vi "Begin.vi"() -> (0 "error out":errorcluster)   [LabVIEW 2013]
doc: "Called before other user functions, this VI is expected to open initial I/O refnums, load in file data, and do all program initialization. Notice that the <B>error out</B> terminal is simply used for data flow. Wiring it to other structures or subVIs ensures that this VI runs first."
uses:
  <vilib>/Rock Robotics/WPI/DriverStation/WPI_DriverStationRobotMode2.ctl
  <vilib>/Rock Robotics/WPI/Joystick/WPI_JoystickDeviceEnum.ctl
  <vilib>/Rock Robotics/SystemInterfaces/DIO/FPGA_DIOPWMChannel.ctl
  <vilib>/Rock Robotics/SystemInterfaces/AI/FPGA_AIGyroChannel.ctl
  <vilib>/Rock Robotics/SystemInterfaces/Typedef/FPGA_TypedefAnalogModuleForGyro.ctl
  <vilib>/Rock Robotics/SystemInterfaces/DIO/FPGA_DIOChannel.ctl
  <vilib>/Rock Robotics/SystemInterfaces/AI/FPGA_AIChannel.ctl
  <vilib>/Rock Robotics/SystemInterfaces/Typedef/FPGA_TypedefAnalogModule.ctl
  <vilib>/Rock Robotics/SystemInterfaces/DIO/FPGA_DIORelayChannel.ctl
  <vilib>/Rock Robotics/SystemInterfaces/Typedef/FPGA_TypedefDigitalModule.ctl
  Robot Global Data.vi
  <vilib>/Rock Robotics/WPI/MotorControl/WPI_MotorControlOpen Talon.vi
panel:
  out "error out 3":errorcluster
  out "error out 2":errorcluster
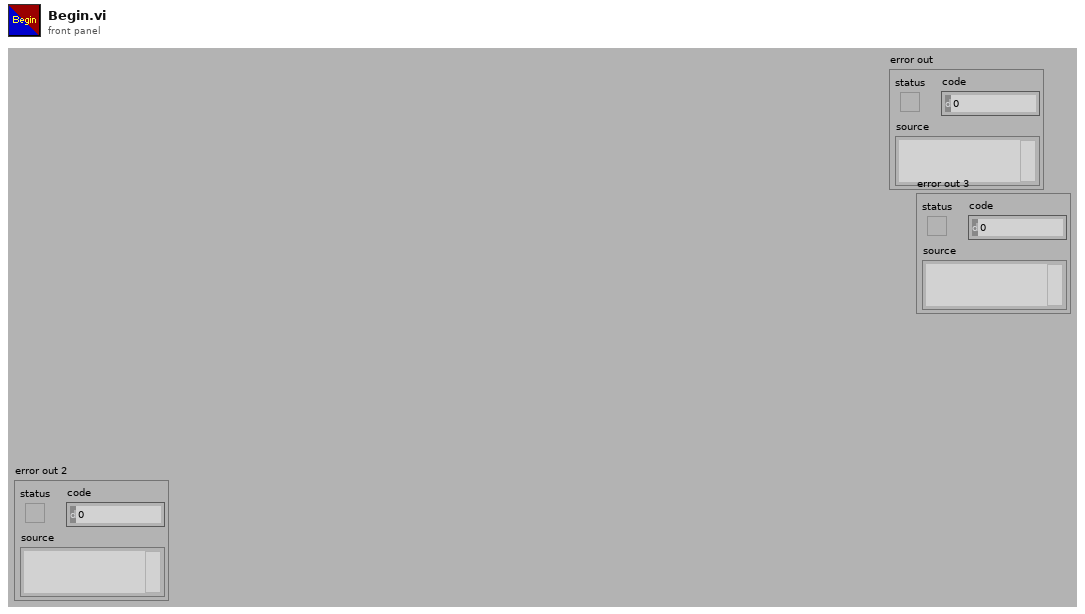
[diagram p1: front panel]
types:
  T1 = typedef "FPGA_TypedefDigitalModule.ctl" = enum16{"Digital Module 1", "Digital Module 2"}
  T2 = typedef "FPGA_DIORelayChannel.ctl" = enum8{"Relay 1", "Relay 2", "Relay 3", "Relay 4", "Relay 5", "Relay 6", "Relay 7", "Relay 8", "Invalid"}
  T3 = typedef "FPGA_DIOChannel.ctl" = enum8{"DIO 1", "DIO 2", "DIO 3", "DIO 4", "DIO 5", "DIO 6", "DIO 7", "DIO 8", "DIO 9", "DIO 10", "DIO 11", "DIO 12", "DIO 13", "DIO 14", "Invalid"}
  T4 = typedef "FPGA_DIOPWMChannel.ctl" = enum8{"PWM 1", "PWM 2", "PWM 3", "PWM 4", "PWM 5", "PWM 6", "PWM 7", "PWM 8", "PWM 9", "PWM 10", "Invalid"}
  T5 = typedef "FPGA_TypedefAnalogModule.ctl" = enum16{"Analog Module 1", "Analog Module 2"}
  T6 = typedef "FPGA_AIChannel.ctl" = enum8{"AI 1", "AI 2", "AI 3", "AI 4", "AI 5", "AI 6", "AI 7", "AI 8", "Invalid"}
  T7 = typedef "WPI_JoystickDeviceEnum.ctl" = enum16{"USB 1", "USB 2", "USB 3", "USB 4", "Kinect 1", "Kinect 2"}
  T8 = typedef "FPGA_TypedefAnalogModuleForGyro.ctl" = enum16{"Analog Module 1"}
  T9 = typedef "FPGA_AIGyroChannel.ctl" = enum8{"AI 1", "AI 2", "Invalid"}
  T10 = typedef "WPI_DriverStationRobotMode2.ctl" = enum16{"Autonomous Disabled", "Autonomous Enabled", "Teleop Disabled", "Teleop Enabled", "Timeout", "Finish", "Test Disabled", "Test Enabled"}
  T11 = typedef "WPI_JoystickDevRef.ctl" = cluster{"Device":T7}
  T12 = typedef "WPI_ServoDeviceRef.ctl" = cluster{"DeviceStatus":errorcluster, "Digital Module":T1, "PWM Channel":T4, "DeadBand":T13}
  T13 = typedef "WPI_PWMDeadband.ctl" = cluster{"Name":string, "maxPositivePwm":i32, "minPositivePwm":i32, "centerPwm":i32, "maxNegativePwm":i32, "minNegativePwm":i32, "angularRange":u16}
  T14 = typedef "WPI_MotorControlDeviceRef.ctl" = cluster{"DeviceStatus":errorcluster, "Type":enum16{"PWM", "CAN"}, "PWM":cluster{"Digital Module":T1, "PWM Channel":T4, "DeadBand":T13}, "CAN":cluster{"Device Number":u8, "Control Mode":T15, "Semaphore":T16, "Max Vout":dbl}, "Invert":bool, "TransformRef":T17, "InvTransformRef":T17}
  T15 = typedef "WPI_CANJaguar_ControlMode.ctl" = enum8{"Percent VBus", "Current", "Speed", "Position", "Voltage"}
  T16 = typedef "Semaphore RefNum" = refnum<k1>
  T17 = typedef "WPI_PWMTransform_ConPane.ctl" = refnum<vi>
  T18 = typedef "WPI_RelayDevRef.ctl" = cluster{"DevStatus":errorcluster, "Relay Channel":T2, "Digital Module":T1, "Relay Direction":T19}
  T19 = typedef "WPI_RelayDirection.ctl" = enum16{"Both directions", "Forward only", "Reverse only"}
  T20 = typedef "WPI_DigitalInputDevRef.ctl" = cluster{"DevStatus":errorcluster, "DIO Channel":T3, "Digital Module":T1}
  T21 = typedef "WPI_AnalogChannelDevRef.ctl" = cluster{"DevStatus":errorcluster, "Analog Module":T5, "Analog Channel":T6}
  T22 = typedef "WPI_GyroDevRef.ctl" = cluster{"DevStatus":errorcluster, "Analog Module":T5, "Analog Channel":T6, "Offset":dbl, "Gain (VoltsPerDegree/Second)":dbl}
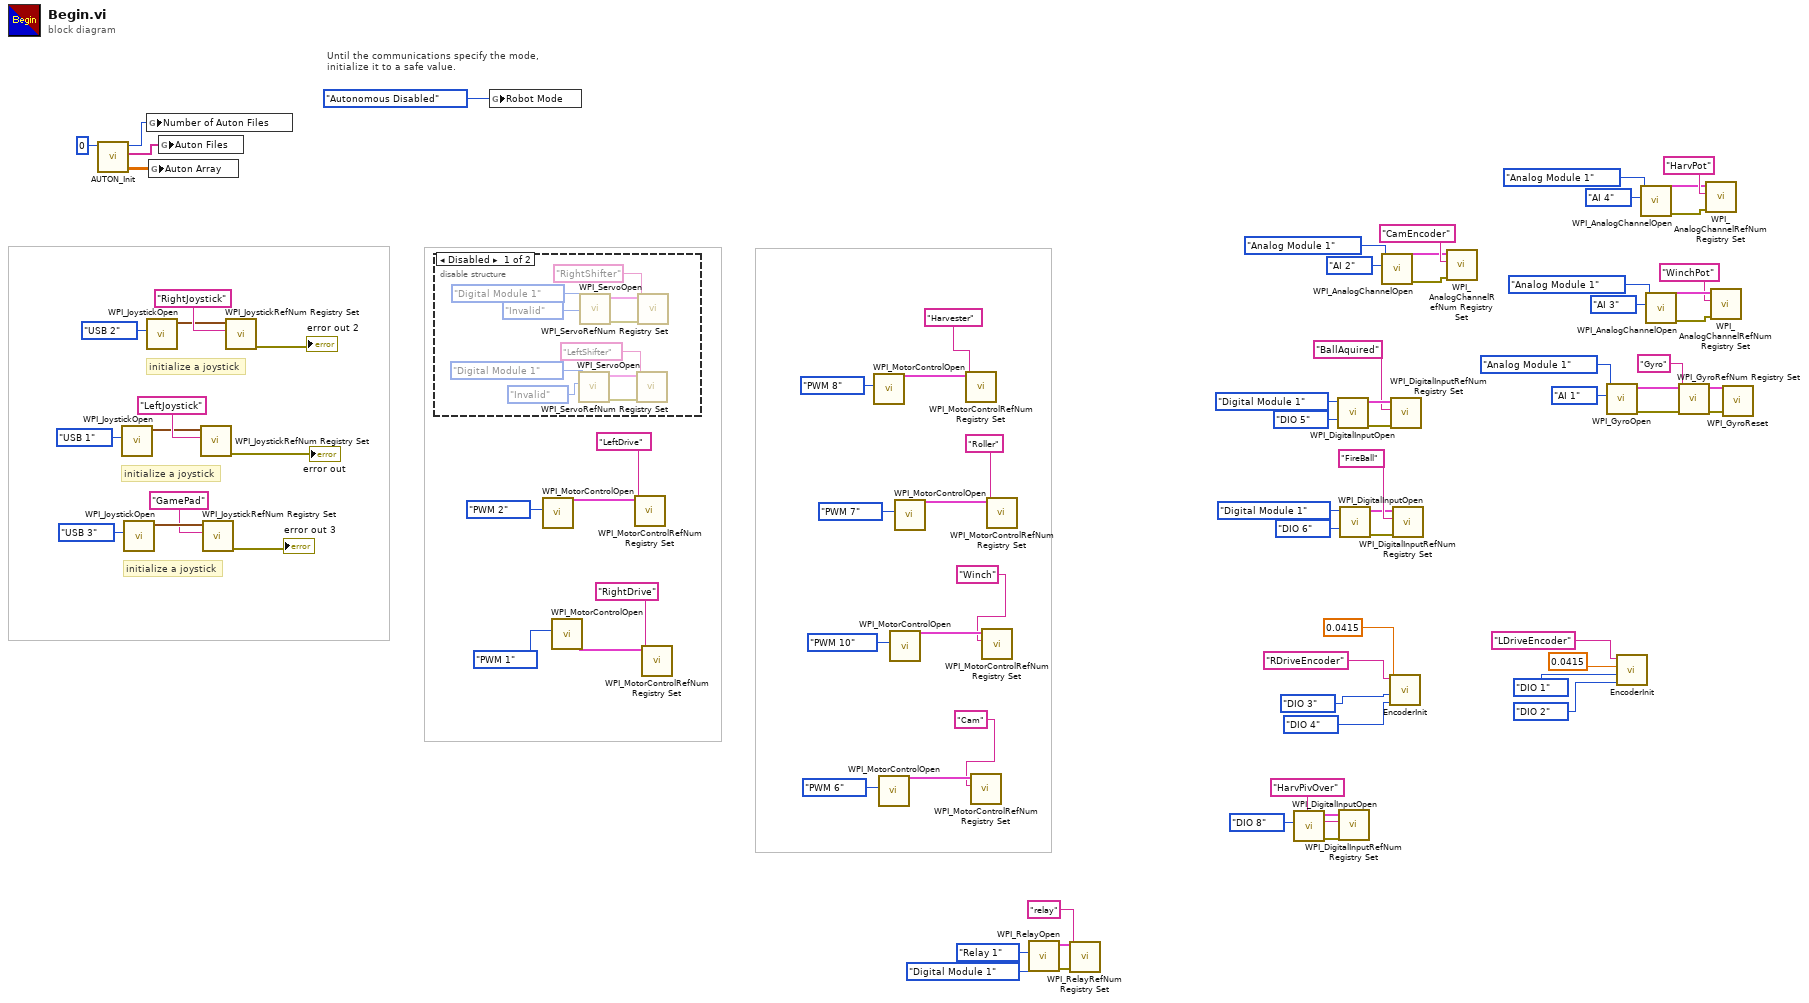
[diagram p0: block diagram]
diagram:
  # "initialize a joystick"
  # "initialize a joystick"
  # "initialize a joystick"
  # "Until the communications specify the mode,\ninitialize it to a safe value."
  n1 = call "AUTON_Init.vi"("Default File"=0) -> ("Auton Array"=w68:dbl[][], "Auton Files"=w67:string[], "Number of Auton Files"=w66:i64)  [unwired: 8 in]
  n2 = call <vilib>:"WPI_JoystickOpen.vi"("JoystickDevice"=WPI_JoystickDeviceEnum."USB 1") -> ("JoystickDevRef"=w82:T11)  [unwired: 10 in]
  n3 = call <vilib>:"WPI_JoystickOpen.vi"("JoystickDevice"=WPI_JoystickDeviceEnum."USB 3") -> ("JoystickDevRef"=w46:T11)  [unwired: 10 in]
  n4 = global write "Robot Global Data.vi" "Number of Auton Files"(w66) -> ()
  n5 = call <vilib>:"WPI_JoystickOpen.vi"("JoystickDevice"=WPI_JoystickDeviceEnum."USB 2") -> ("JoystickDevRef"=w78:T11)  [unwired: 10 in]
  n6 = global write "Robot Global Data.vi" "Auton Array"(w68) -> ()
  n7 = global write "Robot Global Data.vi" "Auton Files"(w67) -> ()
  n8 = call <vilib>:"WPI_JoystickRefNum Registry Set.vi"("refnum name"="LeftJoystick", "JoystickDevRef"=w82) -> ("error out"=→"error out":errorcluster)  [unwired: 8 in, 1 out]
  n9 = call <vilib>:"WPI_JoystickRefNum Registry Set.vi"("refnum name"="GamePad", "JoystickDevRef"=w46) -> ("error out"=→"error out 3":errorcluster)  [unwired: 8 in, 1 out]
  n10 = call <vilib>:"WPI_JoystickRefNum Registry Set.vi"("refnum name"="RightJoystick", "JoystickDevRef"=w78) -> ("error out"=→"error out 2":errorcluster)  [unwired: 8 in, 1 out]
  n11 = disable-structure shown="Disabled" {
    frame Disabled {
      n12 = call <vilib>:"WPI_ServoOpen.vi"("PWM Channel"=FPGA_DIOPWMChannel."Invalid", "Digital Module (Module 1)"=FPGA_TypedefDigitalModule."Digital Module 1") -> ("error out"=w94:errorcluster, "ServoDeviceRef"=w87:T12)  [unwired: 8 in]
      n13 = call <vilib>:"WPI_ServoOpen.vi"("PWM Channel"=FPGA_DIOPWMChannel."Invalid", "Digital Module (Module 1)"=FPGA_TypedefDigitalModule."Digital Module 1") -> ("error out"=w93:errorcluster, "ServoDeviceRef"=w92:T12)  [unwired: 8 in]
      n14 = call <vilib>:"WPI_ServoRefNum Registry Set.vi"("error in (no error)"=w94, "refnum name"="LeftShifter", "ServoDeviceRef"=w87) -> ()  [unwired: 7 in, 2 out]
      n15 = call <vilib>:"WPI_ServoRefNum Registry Set.vi"("error in (no error)"=w93, "refnum name"="RightShifter", "ServoDeviceRef"=w92) -> ()  [unwired: 7 in, 2 out]
    }
    frame Enabled {
    }
  }
  n16 = global write "Robot Global Data.vi" "Robot Mode"(WPI_DriverStationRobotMode2."Autonomous Disabled" ("Robot Mode")) -> ()
  n17 = call-poly <vilib>:"WPI_MotorControlOpen.vi"("PWM Channel"=FPGA_DIOPWMChannel."PWM 2") -> ("MotorControlDeviceRef"=w74:T14)  [unwired: 9 in, 1 out]
  n18 = call-poly <vilib>:"WPI_MotorControlOpen.vi"("PWM Channel"=FPGA_DIOPWMChannel."PWM 1") -> ("MotorControlDeviceRef"=w71:T14)  [unwired: 9 in, 1 out]
  n19 = call <vilib>:"WPI_MotorControlRefNum Registry Set.vi"("refnum name"="LeftDrive", "MotorControlDevRef"=w74) -> ()  [unwired: 8 in, 2 out]
  n20 = call <vilib>:"WPI_MotorControlRefNum Registry Set.vi"("refnum name"="RightDrive", "MotorControlDevRef"=w71) -> ()  [unwired: 8 in, 2 out]
  n21 = call-poly <vilib>:"WPI_MotorControlOpen.vi"("PWM Channel"=FPGA_DIOPWMChannel."PWM 8") -> ("MotorControlDeviceRef"=w64:T14)  [unwired: 9 in, 1 out]
  n22 = call-poly <vilib>:"WPI_MotorControlOpen.vi"("PWM Channel"=FPGA_DIOPWMChannel."PWM 6") -> ("MotorControlDeviceRef"=w28:T14)  [unwired: 9 in, 1 out]
  n23 = call-poly <vilib>:"WPI_MotorControlOpen.vi"("PWM Channel"=FPGA_DIOPWMChannel."PWM 10") -> ("MotorControlDeviceRef"=w30:T14)  [unwired: 9 in, 1 out]
  n24 = call-poly <vilib>:"WPI_MotorControlOpen.vi"("PWM Channel"=FPGA_DIOPWMChannel."PWM 7") -> ("MotorControlDeviceRef"=w62:T14)  [unwired: 9 in, 1 out]
  n25 = call <vilib>:"WPI_MotorControlRefNum Registry Set.vi"("refnum name"="Harvester", "MotorControlDevRef"=w64) -> ()  [unwired: 8 in, 2 out]
  n26 = call <vilib>:"WPI_MotorControlRefNum Registry Set.vi"("refnum name"="Cam", "MotorControlDevRef"=w28) -> ()  [unwired: 8 in, 2 out]
  n27 = call <vilib>:"WPI_MotorControlRefNum Registry Set.vi"("refnum name"="Winch", "MotorControlDevRef"=w30) -> ()  [unwired: 8 in, 2 out]
  n28 = call <vilib>:"WPI_MotorControlRefNum Registry Set.vi"("refnum name"="Roller", "MotorControlDevRef"=w62) -> ()  [unwired: 8 in, 2 out]
  n29 = call <vilib>:"WPI_RelayOpen.vi"("Relay Channel"=FPGA_DIORelayChannel."Relay 1", "Digital Module (Module 1)"=FPGA_TypedefDigitalModule."Digital Module 1") -> ("error out"=w4:errorcluster, "RelayDevRef"=w3:T18)  [unwired: 8 in]
  n30 = call <vilib>:"WPI_RelayRefNum Registry Set.vi"("error in (no error)"=w4, "refnum name"="relay", "RelayDevRef"=w3) -> ()  [unwired: 7 in, 2 out]
  n31 = call <vilib>:"WPI_DigitalInputOpen.vi"("DIO Channel"=FPGA_DIOChannel."DIO 8") -> ("error out"=w32:errorcluster, "DigitalInputDevRef"=w33:T20)  [unwired: 9 in]
  n32 = call <vilib>:"WPI_DigitalInputOpen.vi"("DIO Channel"=FPGA_DIOChannel."DIO 5", "Digital Module (Module 1)"=FPGA_TypedefDigitalModule."Digital Module 1") -> ("error out"=w56:errorcluster, "DigitalInputDevRef"=w55:T20)  [unwired: 8 in]
  n33 = call <vilib>:"WPI_DigitalInputRefNum Registry Set.vi"("error in (no error)"=w32, "refnum name"="HarvPivOver", "DigitalInputDevRef"=w33) -> ()  [unwired: 7 in, 2 out]
  n34 = call <vilib>:"WPI_DigitalInputOpen.vi"("DIO Channel"=FPGA_DIOChannel."DIO 6", "Digital Module (Module 1)"=FPGA_TypedefDigitalModule."Digital Module 1") -> ("error out"=w16:errorcluster, "DigitalInputDevRef"=w17:T20)  [unwired: 8 in]
  n35 = call <vilib>:"WPI_AnalogChannelOpen.vi"("Analog Channel"=FPGA_AIChannel."AI 2", "Analog Module (Module 1)"=FPGA_TypedefAnalogModule."Analog Module 1") -> ("error out"=w22:errorcluster, "AIDeviceRef"=w21:T21)  [unwired: 8 in]
  n36 = call "EncoderInit.vi"("refnum name"="RDriveEncoder", "DistancePerCount"=0.0415, "DIO Channel"=FPGA_DIOChannel."DIO 3", "DIO Channel 2"=FPGA_DIOChannel."DIO 4") -> ()  [unwired: 7 in]
  n37 = call <vilib>:"WPI_DigitalInputRefNum Registry Set.vi"("error in (no error)"=w56, "refnum name"="BallAquired", "DigitalInputDevRef"=w55) -> ()  [unwired: 7 in, 2 out]
  n38 = call <vilib>:"WPI_DigitalInputRefNum Registry Set.vi"("error in (no error)"=w16, "refnum name"="FireBall", "DigitalInputDevRef"=w17) -> ()  [unwired: 7 in, 2 out]
  n39 = call <vilib>:"WPI_AnalogChannelRefNum Registry Set.vi"("error in (no error)"=w22, "refnum name"="CamEncoder", "AIDeviceRef"=w21) -> ()  [unwired: 7 in, 2 out]
  n40 = call <vilib>:"WPI_GyroOpen.vi"("Analog Channel"=FPGA_AIGyroChannel."AI 1", "Analog Module (Module 1)"=FPGA_TypedefAnalogModuleForGyro."Analog Module 1") -> ("error out"=w49:errorcluster, "GyroDevRef"=w59:T22)  [unwired: 7 in, 1 out]
  n41 = call "EncoderInit.vi"("refnum name"="LDriveEncoder", "DistancePerCount"=0.0415, "DIO Channel"=FPGA_DIOChannel."DIO 1", "DIO Channel 2"=FPGA_DIOChannel."DIO 2") -> ()  [unwired: 7 in]
  n42 = call <vilib>:"WPI_AnalogChannelOpen.vi"("Analog Channel"=FPGA_AIChannel."AI 4", "Analog Module (Module 1)"=FPGA_TypedefAnalogModule."Analog Module 1") -> ("error out"=w12:errorcluster, "AIDeviceRef"=w11:T21)  [unwired: 8 in]
  n43 = call <vilib>:"WPI_AnalogChannelOpen.vi"("Analog Channel"=FPGA_AIChannel."AI 3", "Analog Module (Module 1)"=FPGA_TypedefAnalogModule."Analog Module 1") -> ("error out"=w43:errorcluster, "AIDeviceRef"=w44:T21)  [unwired: 8 in]
  n44 = call <vilib>:"WPI_GyroRefNum Registry Set.vi"("error in (no error)"=w49, "refnum name"="Gyro", "GyroDevRef"=w59) -> ("error out"=w50:errorcluster, "GyroDevRef"=w51:T22)  [unwired: 7 in]
  n45 = call <vilib>:"WPI_AnalogChannelRefNum Registry Set.vi"("error in (no error)"=w12, "refnum name"="HarvPot", "AIDeviceRef"=w11) -> ()  [unwired: 7 in, 2 out]
  n46 = call <vilib>:"WPI_AnalogChannelRefNum Registry Set.vi"("error in (no error)"=w43, "refnum name"="WinchPot", "AIDeviceRef"=w44) -> ()  [unwired: 7 in, 2 out]
  n47 = call <vilib>:"WPI_GyroReset.vi"("error in (no error)"=w50, "GyroDevRef"=w51) -> ()  [unwired: 8 in, 2 out]
